vi "Q -- check range -- i -- integer.vi"(4 "upper":i32=99, 6 "lower":i32, 8 "default":i32, 11 "number":i32=11) -> (0 "selector":T1, 2 "in range?":bool=TRUE, 3 "number in range":i32)   [LabVIEW 2021]
uses:
  comparison control.ctl
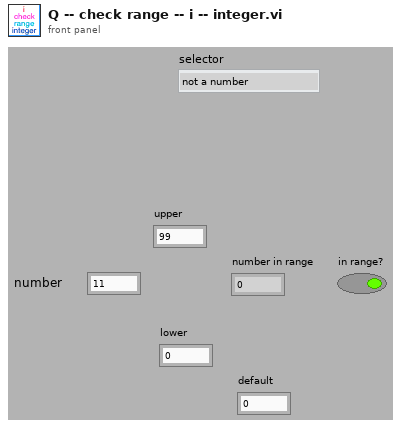
[diagram p1: front panel]
types:
  T1 = typedef "comparison control.ctl" = enum16{"not a number", "above", "in range", "below"}
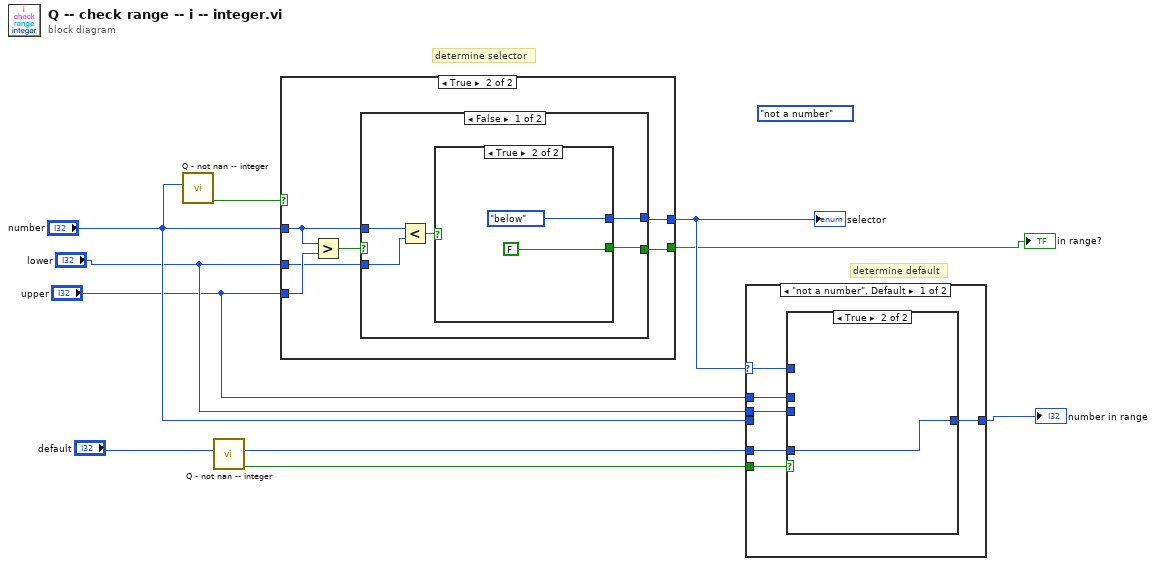
[diagram p0: block diagram]
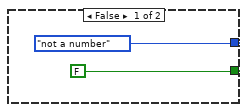
[diagram p5: hidden frame]
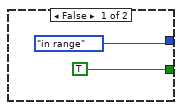
[diagram p6: hidden frame]
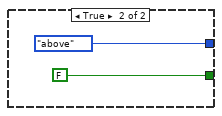
[diagram p7: hidden frame]
diagram:
  (unwired) comparison_control."not a number" ("selector")
  # "determine default"
  # "determine selector"
  n1 = call "Q - not nan -- integer.vi"("Numeric"="number") -> ("Boolean"=w10:bool)  [unwired: 9 in, 1 out]
  n2 = call "Q - not nan -- integer.vi"("Numeric"="default") -> ("Boolean"=w9:bool, "out"=w8:i32)  [unwired: 9 in]
  n3 = case shown="True" w10 {
    tunnel: "upper" -> [_ w17]
    tunnel: "lower" -> [_ w14]
    tunnel: [FALSE w13] -> w1
    tunnel: [comparison_control."not a number" ("selector") w18] -> w2
    tunnel: "number" -> [_ w15]
    frame False {
    }
    frame True {
      n4 = Greater?(x=w15, y=w17) -> (0:w16:bool)
      n5 = case shown="False" w16 {
        tunnel: [w23 comparison_control."above" ("selector")] -> w18
        tunnel: w15 -> [w22 _]
        tunnel: w14 -> [w21 _]
        tunnel: [w19 FALSE] -> w13
        frame False {
          n6 = Less?(x=w22, y=w21) -> (x < y?=w20:bool)
          n7 = case shown="True" w20 {
            tunnel: [comparison_control."in range" ("selector") comparison_control."below" ("selector")] -> w23
            tunnel: [TRUE FALSE] -> w19
            frame False {
            }
            frame True {
            }
          }
        }
        frame True {
        }
      }
    }
  }
  "in range?" <- w1
  "selector" <- w2
  n8 = case shown="\"not a number\", Default" w2 {
    selector: w2 -> [w32 _]
    tunnel: [w34 w43] -> w3
    tunnel: "number" -> [_ w43]
    tunnel: w9 -> [w35 _]
    tunnel: w8 -> [w33 _]
    tunnel: "upper" -> [w31 _]
    tunnel: "lower" -> [w30 _]
    frame "not a number", Default {
      n9 = case shown="True" w35 {
        tunnel: [w38 w42] -> w34
        tunnel: w33 -> [_ w42]
        tunnel: w32 -> [w39 _]
        tunnel: w31 -> [w37 _]
        tunnel: w30 -> [w36 _]
        frame False {
          n10 = case shown="\"not a number\", Default" w39 {
            tunnel: [w40 w41] -> w38
            tunnel: w37 -> [_ w41]
            tunnel: w36 -> [w40 _]
            frame "not a number", Default {
            }
            frame "above" {
            }
          }
        }
        frame True {
        }
      }
    }
    frame "in range" {
    }
  }
  "number in range" <- w3
